vi "Copy Scripting API to Installed Location.vi"(5 "Files Generated by Build":path[](array[path]), 6 "Top Level/Always Included VIs":path[](array[path]), 7 "Destination Path":path, 8 "error in (no error)":errorcluster, 9 "Target Name":string, 10 "Build Specification Name":string, 11 "Project Path":path) -> (0 "error out":errorcluster)   [LabVIEW 2019]
doc: "This VI is called after each run of a build specification. The VI will copy the generated LLB (Engine or System Explorer) into the VeriStand Custom Device folder (...\\Documents\\National Instruments\\NI VeriStand 2013...)."
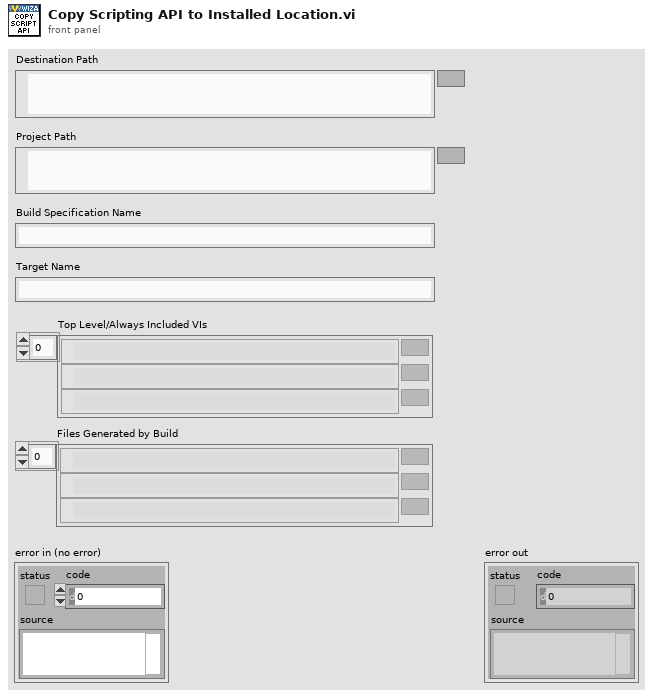
[diagram p1: front panel]
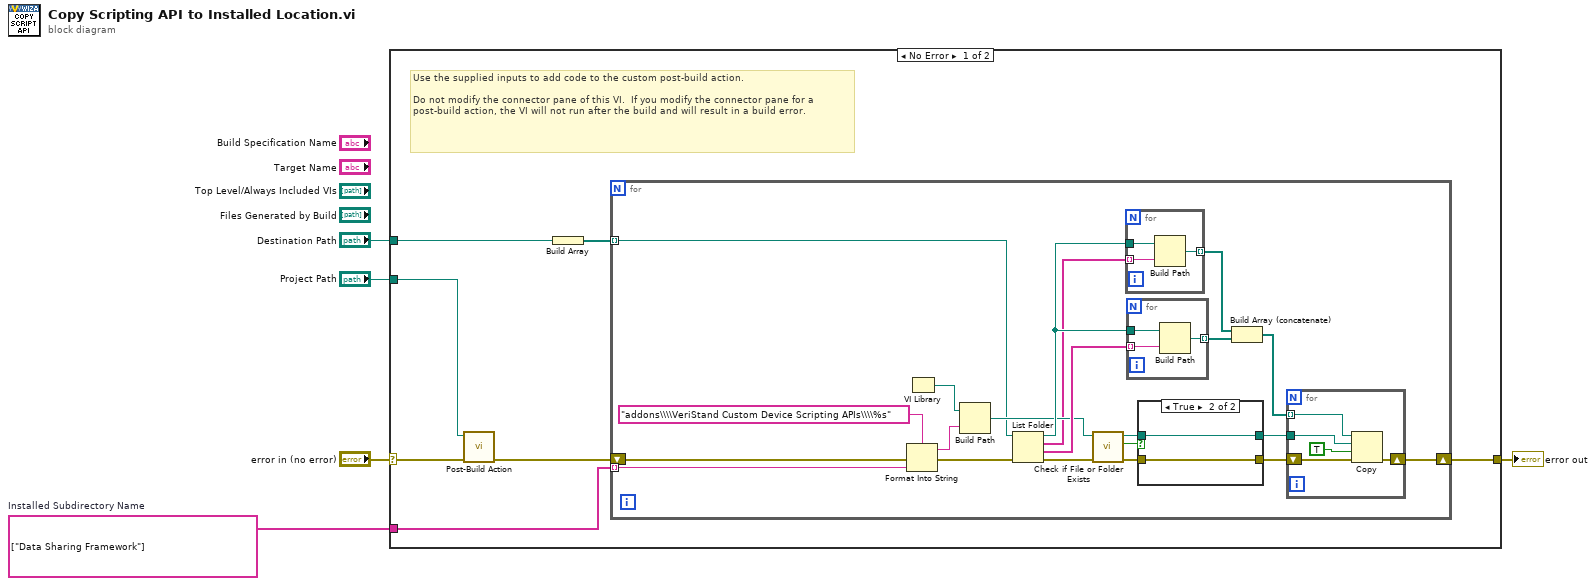
[diagram p0: block diagram]
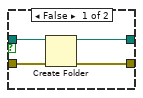
[diagram p2: hidden frame]
diagram:
  w4 = string[] ["Data Sharing Framework"]  # Installed Subdirectory Name
  n1 = case shown="No Error" "error in (no error)" {
    selector: "error in (no error)" -> [w8 w51]
    tunnel: [w11 w51] -> w3
    tunnel: w4 -> [w12 _]
    tunnel: "Destination Path" -> [w9 _]
    tunnel: "Project Path" -> [w6 _]
    frame No Error {
      # "Use the supplied inputs to add code to the custom post-build action.\n\nDo not modify the connector pane of this VI.  If you modify the connector pane for a post-build action, the VI will not run after the build and will result in a build error."
      n2 = call "Post-Build Action.vi"("error in (no error)"=w8, "Project Path"=w6) -> ("error out"=w7:errorcluster)  [unwired: 9 in]
      n3 = Build Array(w9) -> (w10:path[])
      n4 = for {
        tunnel: w12 -> [w19] mode=indexing
        tunnel: w10 -> [w13] mode=indexing
        shift-right: [w14] -> w11
        shift-left: w7 -> [w21]
        n5 = Format Into String(format string="addons\\\\VeriStand Custom Device Scripting APIs\\\\%s" ("name or relative path"), error in=w21, w19) -> (resulting string=w24:string, error out=w20:errorcluster)  [unwired: 1 in]
        n6 = VI Library() -> (path=w15:path)
        n7 = Build Path(base path=w15, name or relative path=w24) -> (appended path=w22:path)
        n8 = List Folder(path=w13, error in=w20) -> (path out=w27:path, filenames=w17:string[], folder names=w28:string[], error out=w25:errorcluster)  [unwired: 2 in]
        n9 = call <vilib>:"Check if File or Folder Exists.vi"("error in (no error)"=w25, "path"=w22) -> ("error out"=w29:errorcluster, "file or folder exists?"=w31:bool, "dup path"=w30:path)  [unwired: 7 in]
        n10 = for {
          tunnel: w17 -> [w49] mode=indexing
          tunnel: w27 -> [w50]
          tunnel: [w48] -> w33 mode=indexing
          n11 = Build Path(base path=w50, name or relative path=w49) -> (appended path=w48:path)
        }
        n12 = for {
          tunnel: w28 -> [w46] mode=indexing
          tunnel: w27 -> [w47]
          tunnel: [w45] -> w26 mode=indexing
          n13 = Build Path(base path=w47, name or relative path=w46) -> (appended path=w45:path)
        }
        n14 = case shown="True" w31 {
          tunnel: w30 -> [w37 w39]
          tunnel: w29 -> [w36 w38]
          tunnel: [w35 w39] -> w16
          tunnel: [w34 w38] -> w18
          frame False {
            n15 = Create Folder(path (use dialog)=w37, error in=w36) -> (created path=w35:path, error out=w34:errorcluster)  [unwired: 1 in, 1 out]
          }
          frame True {
          }
        }
        n16 = Build Array (concatenate)(w33, w26) -> (w32:path[])
        n17 = for {
          tunnel: w32 -> [w41] mode=indexing
          shift-right: [w42] -> w14
          shift-left: w18 -> [w43]
          tunnel: w16 -> [w40]
          n18 = Copy(8:w43, 9:TRUE ("overwrite (F)"), 10:w40, 11:w41) -> (0:w42:errorcluster)  [unwired: 1 in, 2 out]
        }
      }
    }
    frame Error {
    }
  }
  "error out" <- w3
